vi "Excel表格整体转浮点数.vi"(11 "Cam1Light1数据":string[][](array[string])) -> (3 "数组":dbl[][](array[numeric]))   [LabVIEW 2014]
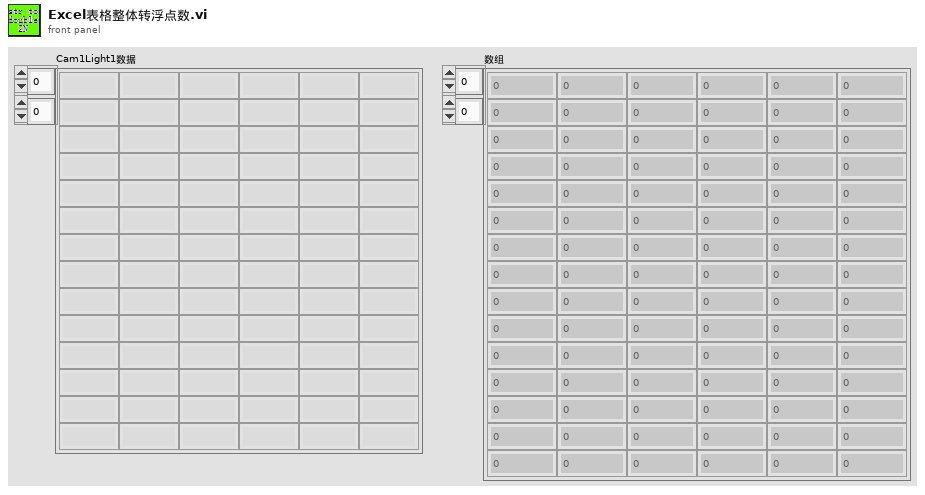
[diagram p1: front panel]
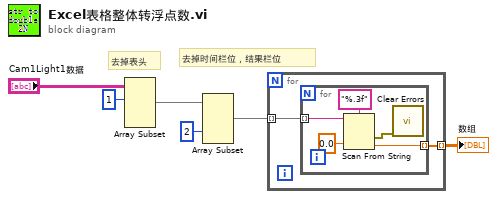
[diagram p0: block diagram]
diagram:
  # "去掉时间栏位，结果栏位"
  # "去掉表头"
  n1 = Array Subset(array="Cam1Light1数据", index (row)=1 ("索引 (行)")) -> (w4:string[][])  [unwired: 3 in]
  n2 = Array Subset(array=w4, index (col)=2 ("索引")) -> (w2:string[][])  [unwired: 3 in]
  n3 = for {
    tunnel: w2 -> [w8] mode=indexing
    tunnel: [w7] -> w1 mode=indexing
    n4 = for {
      tunnel: w8 -> [w13] mode=indexing
      tunnel: [w11] -> w7 mode=indexing
      n5 = Scan From String(format string="%.3f" ("格式字符串"), input string=w13, default 1=0.0 ("默认值 1")) -> (error out=w10:errorcluster, output 1=w11:dbl)  [unwired: 2 in, 2 out]
      n6 = call <vilib>:"Clear Errors.vi"("error in (no error)"=w10) -> ()  [unwired: 5 in, 2 out]
    }
  }
  "数组" <- w1
